vi "Toptica_Commands.vi"() -> ()   [LabVIEW 2011]
panel:
  out "Toptica":T1(array[cluster])=[{"Name"="laser1:label", "Value"="\"640 nm\"", "Type"=4, "Readonly"=TRUE, "comment"=""}, {"Name"="laser1:type", "Value"="\"640nm laser diode\"", "Type"=4, "Readonly"=TRUE, "comment"=""}, {"Name"="laser1:enable", "Value"="#f", "Type"=1, "Readonly"=FALSE, "comment"="prepare emission, can last some seconds"}, {"Name"="laser1:cw", "Value"="#f", "Type"=1, "Readonly"=FALSE, "comment"="laser on, overwrite ext. trigger"}, {"Name"="laser1:ready", "Value"="#t", "Type"=1, "Readonly"=TRUE, "comment"=""}, {"Name"="laser1:fault", "Value"="#f", "Type"=1, "Readonly"=TRUE, "comment"="read status for more information"}, {"Name"="laser1:clip", "Value"="#f", "Type"=1, "Readonly"=TRUE, "comment"="There was an over current, do :reset-clip"}, {"Name"="laser1:reset-clip", "Value"="", "Type"=0, "Readonly"=FALSE, "comment"="reset clip, then reenable"}, {"Name"="laser1:status", "Value"="4097", "Type"=2, "Readonly"=TRUE, "comment"=""}, {"Name"="laser1:status-txt", "Value"="\"AVAILABLE USETTL\"", "Type"=4, "Readonly"=TRUE, "comment"=""}, {"Name"="laser1:level", "Value"="100", "Type"=3, "Readonly"=FALSE, "comment"="Power 0.0-100.0"}, {"Name"="laser1:analog-mode", "Value"="#f", "Type"=1, "Readonly"=FALSE, "comment"="5V= :level, do not apply volatge if #f!"}, {"Name"="laser1:use-ttl", "Value"="#t", "Type"=1, "Readonly"=FALSE, "comment"=""}, {"Name"="laser1:fine:enable", "Value"="#t", "Type"=1, "Readonly"=FALSE, "comment"=""}, {"Name"="laser1:fine:a", "Value"="70.5882", "Type"=3, "Readonly"=FALSE, "comment"=""}, {"Name"="laser1:fine:b", "Value"="30.1961", "Type"=3, "Readonly"=FALSE, "comment"=""}, {"Name"="laser1:delay", "Value"="170", "Type"=2, "Readonly"=FALSE, "comment"="trigger delay 0-255, some ns?"}, {"Name"="laser1:entime", "Value"="1215120", "Type"=2, "Readonly"=TRUE, "comment"="seconds enabled"}, {"Name"="laser1:entime-txt", "Value"="\"337:32:00\"", "Type"=4, "Readonly"=TRUE, "comment"=""}, {"Name"="laser1:ontime", "Value"="120781", "Type"=2, "Readonly"=TRUE, "comment"="seconds on"}, {"Name"="laser1:ontime-txt", "Value"="\"33:33:01\"", "Type"=4, "Readonly"=TRUE, "comment"=""}, {"Name"="laser2:label", "Value"="\"561 nm\"", "Type"=4, "Readonly"=TRUE, "comment"=""}, {"Name"="laser2:type", "Value"="\"FDDL_561\"", "Type"=4, "Readonly"=TRUE, "comment"=""}, {"Name"="laser2:enable", "Value"="#t", "Type"=1, "Readonly"=FALSE, "comment"=""}, {"Name"="laser2:cw", "Value"="#f", "Type"=1, "Readonly"=FALSE, "comment"=""}, {"Name"="laser2:ready", "Value"="#t", "Type"=1, "Readonly"=TRUE, "comment"=""}, {"Name"="laser2:fault", "Value"="#f", "Type"=1, "Readonly"=TRUE, "comment"=""}, {"Name"="laser2:clip", "Value"="#f", "Type"=1, "Readonly"=TRUE, "comment"=""}, {"Name"="laser2:status", "Value"="4099", "Type"=2, "Readonly"=TRUE, "comment"=""}, {"Name"="laser2:status-txt", "Value"="\"AVAILABLE ENABLED USETTL\"", "Type"=4, "Readonly"=TRUE, "comment"=""}, {"Name"="laser2:level", "Value"="100", "Type"=2, "Readonly"=FALSE, "comment"=""}, {"Name"="laser2:analog-mode", "Value"="#f", "Type"=1, "Readonly"=FALSE, "comment"=""}, {"Name"="laser2:use-ttl", "Value"="#t", "Type"=1, "Readonly"=FALSE, "comment"=""}, {"Name"="laser2:fine:enable", "Value"="#t", "Type"=1, "Readonly"=FALSE, "comment"=""}, {"Name"="laser2:fine:a", "Value"="36.8627", "Type"=3, "Readonly"=FALSE, "comment"=""}, {"Name"="laser2:fine:b", "Value"="3.52941", "Type"=3, "Readonly"=FALSE, "comment"=""}, {"Name"="laser2:delay", "Value"="170", "Type"=2, "Readonly"=FALSE, "comment"=""}, {"Name"="laser2:entime", "Value"="782372", "Type"=2, "Readonly"=TRUE, "comment"=""}, {"Name"="laser2:entime-txt", "Value"="\"217:19:32\"", "Type"=4, "Readonly"=TRUE, "comment"=""}, {"Name"="laser2:ontime", "Value"="178489", "Type"=4, "Readonly"=TRUE, "comment"=""}, {"Name"="laser2:ontime-txt", "Value"="\"49:34:49\"", "Type"=0, "Readonly"=TRUE, "comment"=""}, {"Name"="laser2:shg:temp", "Value"="29.102 -> 29.1", "Type"=4, "Readonly"=FALSE, "comment"="read and set"}, {"Name"="laser3:label", "Value"="\"488 nm\"", "Type"=4, "Readonly"=TRUE, "comment"=""}, {"Name"="laser3:type", "Value"="\"488nm laser diode\"", "Type"=4, "Readonly"=TRUE, "comment"=""}, {"Name"="laser3:enable", "Value"="#t", "Type"=1, "Readonly"=FALSE, "comment"=""}, {"Name"="laser3:cw", "Value"="#f", "Type"=1, "Readonly"=FALSE, "comment"=""}, {"Name"="laser3:ready", "Value"="#t", "Type"=1, "Readonly"=TRUE, "comment"=""}, {"Name"="laser3:fault", "Value"="#f", "Type"=1, "Readonly"=TRUE, "comment"=""}, {"Name"="laser3:clip", "Value"="#f", "Type"=1, "Readonly"=TRUE, "comment"=""}, {"Name"="laser3:status", "Value"="4099", "Type"=2, "Readonly"=TRUE, "comment"=""}, {"Name"="laser3:status-txt", "Value"="\"AVAILABLE ENABLED USETTL\"", "Type"=4, "Readonly"=TRUE, "comment"=""}, {"Name"="laser3:level", "Value"="100", "Type"=3, "Readonly"=FALSE, "comment"=""}, {"Name"="laser3:analog-mode", "Value"="#f", "Type"=1, "Readonly"=FALSE, "comment"=""}, {"Name"="laser3:use-ttl", "Value"="#t", "Type"=1, "Readonly"=FALSE, "comment"=""}, {"Name"="laser3:fine:enable", "Value"="#t", "Type"=1, "Readonly"=FALSE, "comment"=""}, {"Name"="laser3:fine:a", "Value"="70.1961", "Type"=3, "Readonly"=FALSE, "comment"=""}, {"Name"="laser3:fine:b", "Value"="10.1961", "Type"=3, "Readonly"=FALSE, "comment"=""}, {"Name"="laser3:delay", "Value"="170", "Type"=2, "Readonly"=FALSE, "comment"=""}, {"Name"="laser3:entime", "Value"="1247813", "Type"=2, "Readonly"=TRUE, "comment"=""}, {"Name"="laser3:entime-txt", "Value"="\"346:36:53\"", "Type"=4, "Readonly"=TRUE, "comment"=""}, {"Name"="laser3:ontime", "Value"="211459", "Type"=2, "Readonly"=TRUE, "comment"=""}, {"Name"="laser3:ontime-txt", "Value"="\"58:44:19\"", "Type"=4, "Readonly"=TRUE, "comment"=""}, {"Name"="laser4:label", "Value"="\"405 nm\"", "Type"=4, "Readonly"=TRUE, "comment"=""}, {"Name"="laser4:type", "Value"="\"405nm laser diode\"", "Type"=4, "Readonly"=TRUE, "comment"=""}, {"Name"="laser4:enable", "Value"="#t", "Type"=1, "Readonly"=FALSE, "comment"=""}, {"Name"="laser4:cw", "Value"="#f", "Type"=1, "Readonly"=FALSE, "comment"=""}, {"Name"="laser4:ready", "Value"="#t", "Type"=1, "Readonly"=TRUE, "comment"=""}, {"Name"="laser4:fault", "Value"="#f", "Type"=1, "Readonly"=TRUE, "comment"=""}, {"Name"="laser4:clip", "Value"="#f", "Type"=1, "Readonly"=TRUE, "comment"=""}, {"Name"="laser4:status", "Value"="4099", "Type"=2, "Readonly"=TRUE, "comment"=""}, {"Name"="laser4:status-txt", "Value"="\"AVAILABLE ENABLED USETTL\"", "Type"=4, "Readonly"=TRUE, "comment"=""}, {"Name"="laser4:level", "Value"="99.8779", "Type"=3, "Readonly"=FALSE, "comment"=""}, {"Name"="laser4:analog-mode", "Value"="#f", "Type"=1, "Readonly"=FALSE, "comment"=""}, {"Name"="laser4:use-ttl", "Value"="#t", "Type"=1, "Readonly"=FALSE, "comment"=""}, {"Name"="laser4:fine:enable", "Value"="#t", "Type"=1, "Readonly"=FALSE, "comment"=""}, {"Name"="laser4:fine:a", "Value"="70.1961", "Type"=3, "Readonly"=FALSE, "comment"=""}, {"Name"="laser4:fine:b", "Value"="10.1961", "Type"=3, "Readonly"=FALSE, "comment"=""}, {"Name"="laser4:delay", "Value"="170", "Type"=2, "Readonly"=FALSE, "comment"=""}, {"Name"="laser4:entime", "Value"="1443557", "Type"=2, "Readonly"=TRUE, "comment"=""}, {"Name"="laser4:entime-txt", "Value"="\"400:59:17\"", "Type"=4, "Readonly"=TRUE, "comment"=""}, {"Name"="laser4:ontime", "Value"="135946", "Type"=2, "Readonly"=TRUE, "comment"=""}, {"Name"="laser4:ontime-txt", "Value"="\"37:45:46\"", "Type"=4, "Readonly"=TRUE, "comment"=""}, {"Name"="all:enable", "Value"="#f", "Type"=1, "Readonly"=FALSE, "comment"="enable all lasers"}, {"Name"="all:enable-led", "Value"="#t", "Type"=1, "Readonly"=TRUE, "comment"="equal to emission led"}, {"Name"="all:cw", "Value"="#f", "Type"=1, "Readonly"=FALSE, "comment"="switch on all lasers"}, {"Name"="all:analog-mode", "Value"="#f", "Type"=1, "Readonly"=FALSE, "comment"=""}, {"Name"="all:use-ttl", "Value"="#t", "Type"=1, "Readonly"=FALSE, "comment"="digital for all laser"}, {"Name"="all:ttl-active-high", "Value"="#t", "Type"=1, "Readonly"=FALSE, "comment"="#t=5V=On"}, {"Name"="all:ttl-master-mode", "Value"="#f", "Type"=1, "Readonly"=FALSE, "comment"="all lasers on trigger on line 1"}, {"Name"="all:digital-over-analog", "Value"="#t", "Type"=1, "Readonly"=FALSE, "comment"="? Comperator?"}, {"Name"="all:ready", "Value"="#t", "Type"=1, "Readonly"=TRUE, "comment"=""}, {"Name"="all:fault", "Value"="#f", "Type"=1, "Readonly"=TRUE, "comment"="#t=at least one fault"}, {"Name"="all:reset-clip", "Value"="", "Type"=0, "Readonly"=FALSE, "comment"="reset all laser clips"}, {"Name"="all:store-config", "Value"="", "Type"=0, "Readonly"=FALSE, "comment"="store: level, cw enable, trigger, fine.."}, {"Name"="tec-d:enable", "Value"="#t", "Type"=1, "Readonly"=FALSE, "comment"="tec for brag grating"}, {"Name"="tec-d:status", "Value"="7", "Type"=2, "Readonly"=TRUE, "comment"=""}, {"Name"="tec-d:status-txt", "Value"="\"ENABLED TEMPOK HEATING\"", "Type"=4, "Readonly"=TRUE, "comment"=""}, {"Name"="tec-d:fault", "Value"="#f", "Type"=1, "Readonly"=TRUE, "comment"=""}, {"Name"="tec-d:temp", "Value"="31.949 -> 32", "Type"=3, "Readonly"=TRUE, "comment"=">stable, with low power"}, {"Name"="tec-l:enable", "Value"="#t", "Type"=1, "Readonly"=FALSE, "comment"="tec for laserhead"}, {"Name"="tec-l:status", "Value"="7", "Type"=2, "Readonly"=TRUE, "comment"=""}, {"Name"="tec-l:status-txt", "Value"="\"ENABLED TEMPOK HEATING\"", "Type"=4, "Readonly"=TRUE, "comment"=""}, {"Name"="tec-l:fault", "Value"="#f", "Type"=1, "Readonly"=TRUE, "comment"=""}, {"Name"="tec-l:temp", "Value"="25.031 -> 25", "Type"=3, "Readonly"=TRUE, "comment"="set?"}, {"Name"="dx5100:serial-number", "Value"="\"#S406 14.04.2014\"", "Type"=4, "Readonly"=TRUE, "comment"=""}, {"Name"="dx5100:fw-ver", "Value"="\"07/20/15 10:21:36 DX5100.346\"", "Type"=4, "Readonly"=TRUE, "comment"=""}, {"Name"="tec-c:enable", "Value"="#t", "Type"=1, "Readonly"=FALSE, "comment"="tec for shg"}, {"Name"="tec-c:status", "Value"="7", "Type"=2, "Readonly"=TRUE, "comment"=""}, {"Name"="tec-c:status-txt", "Value"="\"ENABLED TEMPOK HEATING\"", "Type"=4, "Readonly"=TRUE, "comment"=""}, {"Name"="tec-c:temp", "Value"="29.1013 -> 29.1", "Type"=3, "Readonly"=FALSE, "comment"="optimised for efficency!"}, {"Name"="tec-c:current", "Value"="0", "Type"=3, "Readonly"=TRUE, "comment"=""}, {"Name"="tec-c:voltage", "Value"="0.000143536", "Type"=3, "Readonly"=TRUE, "comment"=""}, {"Name"="tec-c:temp-min", "Value"="18", "Type"=3, "Readonly"=FALSE, "comment"=""}, {"Name"="tec-c:temp-max", "Value"="55", "Type"=3, "Readonly"=FALSE, "comment"=""}, {"Name"="tec-c:kp", "Value"="0.3", "Type"=3, "Readonly"=FALSE, "comment"="0.3"}, {"Name"="tec-c:ki", "Value"="0.1", "Type"=3, "Readonly"=FALSE, "comment"="0.1"}, {"Name"="tec-c:kd", "Value"="0", "Type"=3, "Readonly"=FALSE, "comment"="0"}, {"Name"="tec-c:calibration", "Value"="(#f 0.00110459 0.00023545 1.03481e-07 0 0 0)", "Type"=4, "Readonly"=TRUE, "comment"="thermistor (#f 0.00110459 0.00023545 1.03481e-07 0 0 0)"}, {"Name"="tec-p:enable", "Value"="#t", "Type"=1, "Readonly"=FALSE, "comment"="tec 1122 Diode"}, {"Name"="tec-p:status", "Value"="11", "Type"=2, "Readonly"=TRUE, "comment"=""}, {"Name"="tec-p:status-txt", "Value"="\"ENABLED TEMPOK COOLING\"", "Type"=4, "Readonly"=TRUE, "comment"=""}, {"Name"="tec-p:temp", "Value"="18.0015 -> 18", "Type"=3, "Readonly"=FALSE, "comment"=""}, {"Name"="tec-p:current", "Value"="0.169922", "Type"=3, "Readonly"=TRUE, "comment"=""}, {"Name"="tec-p:voltage", "Value"="0.000159429", "Type"=3, "Readonly"=TRUE, "comment"=""}, {"Name"="tec-p:temp-min", "Value"="15", "Type"=3, "Readonly"=FALSE, "comment"=""}, {"Name"="tec-p:temp-max", "Value"="35", "Type"=3, "Readonly"=FALSE, "comment"=""}, {"Name"="tec-p:kp", "Value"="0.3", "Type"=3, "Readonly"=FALSE, "comment"=""}, {"Name"="tec-p:ki", "Value"="0.1", "Type"=3, "Readonly"=FALSE, "comment"=""}, {"Name"="tec-p:kd", "Value"="0", "Type"=3, "Readonly"=FALSE, "comment"=""}, {"Name"="tec-p:calibration", "Value"="(#f 0.00110459 0.00023545 1.03481e-07 0 0 0)", "Type"=4, "Readonly"=TRUE, "comment"=""}, {"Name"="powermon:cal", "Value"="0", "Type"=3, "Readonly"=TRUE, "comment"=""}, {"Name"="powermon:cal-udelay", "Value"="0", "Type"=2, "Readonly"=FALSE, "comment"="us delay for slow sensors"}, {"Name"="powermon:signal", "Value"="21", "Type"=3, "Readonly"=TRUE, "comment"="used for optimization"}, {"Name"="powermon:signal-source", "Value"="\"int\"", "Type"=4, "Readonly"=FALSE, "comment"="\"int\"=Diode, \"fiber\"=?, \"cal\"=SMB port; auch \"int-na\" und \"fiber-na\" ohne autogain"}, {"Name"="interlock", "Value"="#f", "Type"=1, "Readonly"=TRUE, "comment"=""}, {"Name"="base-temp", "Value"="'Error -16'", "Type"=3, "Readonly"=TRUE, "comment"=""}, {"Name"="buzzer:welcome", "Value"="\" \"", "Type"=4, "Readonly"=TRUE, "comment"=""}, {"Name"="buzzer:play", "Value"="\"A C E F\"", "Type"=5, "Readonly"=FALSE, "comment"=""}, {"Name"="tan", "Value"="0", "Type"=2, "Readonly"=TRUE, "comment"=""}, {"Name"="uptime", "Value"="2269207", "Type"=0, "Readonly"=TRUE, "comment"="seconds"}, {"Name"="uptime-txt", "Value"="\"630:20:07\"", "Type"=4, "Readonly"=TRUE, "comment"=""}, {"Name"="time", "Value"="\"2017-03-20 16:34:29\"", "Type"=4, "Readonly"=TRUE, "comment"=""}, {"Name"="fw-ver", "Value"="\"1.0.0.7\"", "Type"=4, "Readonly"=TRUE, "comment"=""}, {"Name"="decof-ver", "Value"="\"3.1.1476\"", "Type"=4, "Readonly"=TRUE, "comment"=""}, {"Name"="serial-number", "Value"="\"iCHROME_CLE_TILL_Prototyp1\"", "Type"=4, "Readonly"=TRUE, "comment"=""}, {"Name"="system-type", "Value"="\"MLE-Young\"", "Type"=4, "Readonly"=TRUE, "comment"=""}, {"Name"="system-model", "Value"="\"DDDD\"", "Type"=4, "Readonly"=TRUE, "comment"=""}, {"Name"="system-label", "Value"="\"\"", "Type"=4, "Readonly"=FALSE, "comment"=""}, {"Name"="ul", "Value"="3", "Type"=2, "Readonly"=TRUE, "comment"="user level, std=3 lower= more access"}, {"Name"="net-conf:ip-addr", "Value"="\"192.168.2.2\"", "Type"=4, "Readonly"=TRUE, "comment"=""}, {"Name"="net-conf:net-mask", "Value"="\"255.255.255.0\"", "Type"=4, "Readonly"=TRUE, "comment"=""}, {"Name"="net-conf:mac-addr", "Value"="\"00:0C:C6:7F:02:4B\"", "Type"=4, "Readonly"=TRUE, "comment"=""}, {"Name"="net-conf:dhcp", "Value"="#f", "Type"=1, "Readonly"=TRUE, "comment"=""}, {"Name"="net-conf:set-dhcp", "Value"="", "Type"=0, "Readonly"=FALSE, "comment"="enable dhcp"}, {"Name"="net-conf:set-ip", "Value"="", "Type"=6, "Readonly"=FALSE, "comment"="\"192.168.2.1\" \"255.255.255.0\" disable dhcp"}, {"Name"="net-conf:apply", "Value"="", "Type"=0, "Readonly"=FALSE, "comment"="apply dhcp change = loose connection!"}, {"Name"="net-conf:cmd-port", "Value"="50000", "Type"=2, "Readonly"=TRUE, "comment"=""}, {"Name"="net-conf:mon-port", "Value"="0", "Type"=2, "Readonly"=TRUE, "comment"=""}, {"Name"="echo", "Value"="#t", "Type"=1, "Readonly"=FALSE, "comment"="surpress echo"}, {"Name"="script:boot:busy", "Value"="#f", "Type"=1, "Readonly"=TRUE, "comment"=""}, {"Name"="script:boot:size", "Value"="52", "Type"=2, "Readonly"=TRUE, "comment"=""}, {"Name"="script:console:busy", "Value"="#f", "Type"=1, "Readonly"=TRUE, "comment"=""}, {"Name"="script:console:size", "Value"="0", "Type"=2, "Readonly"=TRUE, "comment"=""}, {"Name"="script:misc:busy", "Value"="#f", "Type"=1, "Readonly"=TRUE, "comment"=""}, {"Name"="script:misc:size", "Value"="5532", "Type"=2, "Readonly"=TRUE, "comment"=""}] {"Type" items=["command noarg", "parameter bool", "parameter int", "parameter real", "parameter string", "command 1string", "command 2string", ""]}
  in  "L1 commands":u16(ring) items=["exec", "param-ref", "param-gsv", "param-disp", "param-set!"]
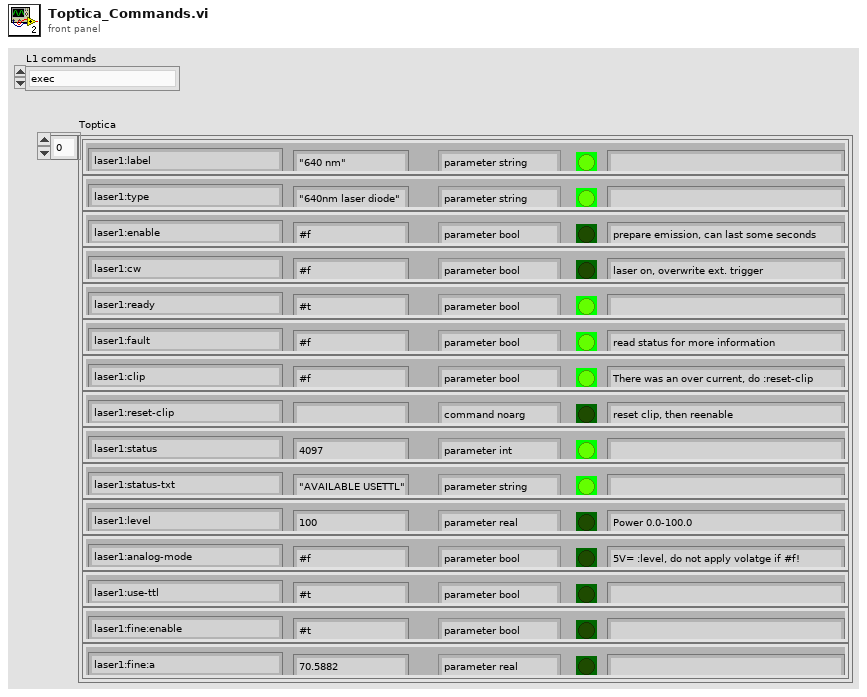
[diagram p1: front panel]
types:
  T1 = cluster{"Name":string, "Value":string, "Type":u16, "Readonly":bool, "comment":string}[]
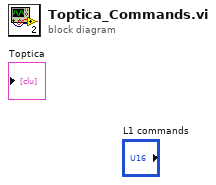
[diagram p0: block diagram]
diagram:
